vi "ql2_term_build.vi"(9 "options (key,val)":string[][](array[string]), 10 "args":string[](array[string]), 11 "term_type":T1) -> (3 "query":string)   [LabVIEW 2017, in "rethinkdb.lvlib"]
uses:
  rethinkdb.lvlib
  ql2_term.ctl
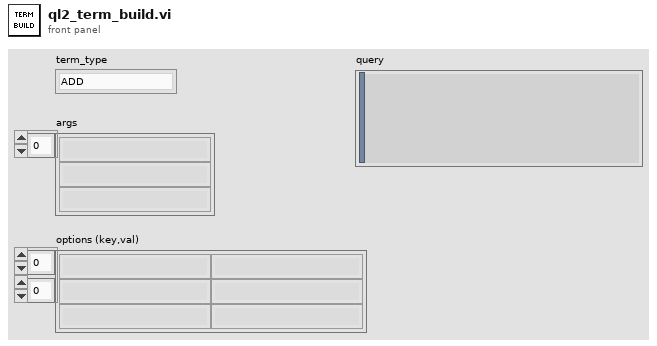
[diagram p1: front panel]
types:
  T1 = typedef "rethinkdb.lvlib/ql2_term.ctl" = enum8{"ADD", "AND", "APPEND", "APRIL", "ARGS", "ASC", "AUGUST", "AVG", "BETWEEN", "BETWEEN_DEPRECATED", "BINARY", "BIT_AND", "BIT_NOT", "BIT_OR", "BIT_SAL", "BIT_SAR", "BIT_XOR", "BRACKET", "BRANCH", "CEIL", "CHANGES", "CHANGE_AT", "CIRCLE", "COERCE_TO", "CONCAT_MAP", "CONFIG", "CONTAINS", "COUNT", "DATE", "DATUM", "DAY", "DAY_OF_WEEK", "DAY_OF_YEAR", "DB", "DB_CREATE", "DB_DROP", "DB_LIST", "DECEMBER", "DEFAULT", "DELETE", "DELETE_AT", "DESC", "DIFFERENCE", "DISTANCE", "DISTINCT", "DIV", "DOWNCASE", "DURING", "EPOCH_TIME", "EQ", "EQ_JOIN", "ERROR", "FEBRUARY", "FILL", "FILTER", "FLOOR", "FOLD", "FOR_EACH", "FRIDAY", "FUNC", "FUNCALL", "GE", "GEOJSON", "GET", "GET_ALL", "GET_FIELD", "GET_INTERSECTING", "GET_NEAREST", "GET_WRITE_HOOK", "GRANT", "GROUP", "GT", "HAS_FIELDS", "HOURS", "HTTP", "IMPLICIT_VAR", "INCLUDES", "INDEX_CREATE", "INDEX_DROP", "INDEX_LIST", "INDEX_RENAME", "INDEX_STATUS", "INDEX_WAIT", "INFO", "INNER_JOIN", "INSERT", "INSERT_AT", "INTERSECTS", "IN_TIMEZONE", "ISO8601", "IS_EMPTY", "JANUARY", "JAVASCRIPT", "JSON", "JULY", "JUNE", "KEYS", "LE", "LIMIT", "LINE", "LITERAL", "LT", "MAKE_ARRAY", "MAKE_OBJ", "MAP", "MARCH", "MATCH", "MAX", "MAXVAL", "MAY", "MERGE", "MIN", "MINUTES", "MINVAL", "MOD", "MONDAY", "MONTH", "MUL", "NE", "NOT", "NOVEMBER", "NOW", "NTH", "OBJECT", "OCTOBER", "OFFSETS_OF", "OR", "ORDER_BY", "OUTER_JOIN", "PLUCK", "POINT", "POLYGON", "POLYGON_SUB", "PREPEND", "RANDOM", "RANGE", "REBALANCE", "RECONFIGURE", "REDUCE", "REPLACE", "ROUND", "SAMPLE", "SATURDAY", "SECONDS", "SEPTEMBER", "SET_DIFFERENCE", "SET_INSERT", "SET_INTERSECTION", "SET_UNION", "SET_WRITE_HOOK", "SKIP", "SLICE", "SPLICE_AT", "SPLIT", "STATUS", "SUB", "SUM", "SUNDAY", "SYNC", "TABLE", "TABLE_CREATE", "TABLE_DROP", "TABLE_LIST", "THURSDAY", "TIME", "TIMEZONE", "TIME_OF_DAY", "TO_EPOCH_TIME", "TO_GEOJSON", "TO_ISO8601", "TO_JSON_STRING", "TUESDAY", "TYPE_OF", "UNGROUP", "UNION", "UPCASE", "UPDATE", "UUID", "VALUES", "VAR", "WAIT", "WEDNESDAY", "WITHOUT", "WITH_FIELDS", "YEAR", "ZIP", "invalid"}
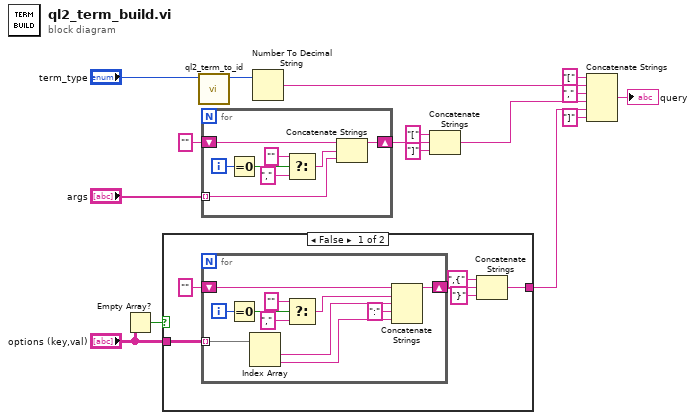
[diagram p0: block diagram]
diagram:
  n1 = Empty Array?(array="options (key,val)") -> (empty?=w3:bool)
  n2 = case shown="False" w3 {
    tunnel: "options (key,val)" -> [w21 _]
    tunnel: [w19 _] -> w8
    frame False {
      n3 = for {
        tunnel: w21 -> [w26] mode=indexing
        shift-right: [w28] -> w20
        shift-left: "" -> [w33]
        i -> [w32]
        n4 = Equal To 0?(x=w32) -> (x = 0?=w31:bool)
        n5 = Index Array(array=w26) -> (element #1=w25:string, element #2=w23:string)  [unwired: 2 in]
        n6 = Select(t="", s=w31, f=",") -> (s? t:f=w27:string)
        n7 = Concatenate Strings(w33, w27, w25, ":" ("string"), w23) -> (w28:string)
      }
      n8 = Concatenate Strings(",{" ("string"), w20, "}" ("string")) -> (w19:string)
    }
    frame True {
    }
  }
  n9 = call "ql2_term_to_id.vi"("term_type"="term_type") -> ("id"=w1:u32)  [unwired: 9 in, 1 out]
  n10 = for {
    tunnel: "args" -> [w34] mode=indexing
    shift-right: [w36] -> w13
    shift-left: "" -> [w41]
    i -> [w40]
    n11 = Equal To 0?(x=w40) -> (x = 0?=w39:bool)
    n12 = Select(t="", s=w39, f=",") -> (s? t:f=w35:string)
    n13 = Concatenate Strings(w41, w35, w34) -> (w36:string)
  }
  n14 = Number To Decimal String(number=w1) -> (decimal integer string=w16:string)  [unwired: 1 in]
  n15 = Concatenate Strings("[" ("string"), w13, "]" ("string")) -> (w7:string)
  n16 = Concatenate Strings("[" ("string"), w16, "," ("string"), w7, w8, "]" ("string")) -> (→"query":string)
